vi "PH_OceanOpticsSpectrometer.ProcCases.vi"(0 "i ref in":refnum<vi>, 1 "selector":string, 2 "Data":T1, 3 "call cluster":T2={"Object"="", "Selector"="", "CallType"=enum."synchronous", "Async Object"="", "Async Selector"="", "Data Descriptor"="", "Data"=[], "Error #"=0, "Expire"=0}, 5 "error in (no error)":errorcluster) -> (14 "i ref out":refnum<vi>, 17 "answer cluster":T2={"Object"="", "Selector"="", "CallType"=enum."synchronous", "Async Object"="", "Async Selector"="", "Data Descriptor"="", "Data"=[], "Error #"=0, "Expire"=0}, 19 "error out":errorcluster)   [LabVIEW 2014, in "PH_OceanOpticsSpectrometer.lvlib"]
doc: "This method is called by a process from within the default case in the event loop. The methods of a class that are linked to events will be called from THIS method. Add your code here."
uses:
  PH_OceanOpticsSpectrometer.lvlib
  CS_Core/CSSystem/CoreDefs/CoreDefs.call_type.ctl
  CS_Core/BaseProcess/BaseProcess.descriptor string definition.ctl
  CS_Core/CSSystem/CoreDefs/CoreDefs.rawDataType.ctl
  CS_Core/CSSystem/CoreLib/CoreLib.byte array 2 short.vi
  CS_Core/CSSystem/CoreLib/CoreLib.string 2 byte array.vi
  CS_Core/CSSystem/CoreLib/CoreLib.byte array 2 double.vi
  CS_Core/BaseProcess/BaseProcess.lvlib
  CS_Core/CSSystem/CoreLib/CoreLib.lvlib
  CS_Core/CSSystem/CSSystemLib/CSSystemLib.lvlib
  CS_Core/CAEObj/CAEObj.lvlib
  PH_Basics/PH_PSDBWriter/PH_PSDBWriter.lvlib
  PH_Basics/PH_Common/PH_Common.lvlib
  PH_Basics/PH_StatusHandler/PH_StatusHandler.lvlib
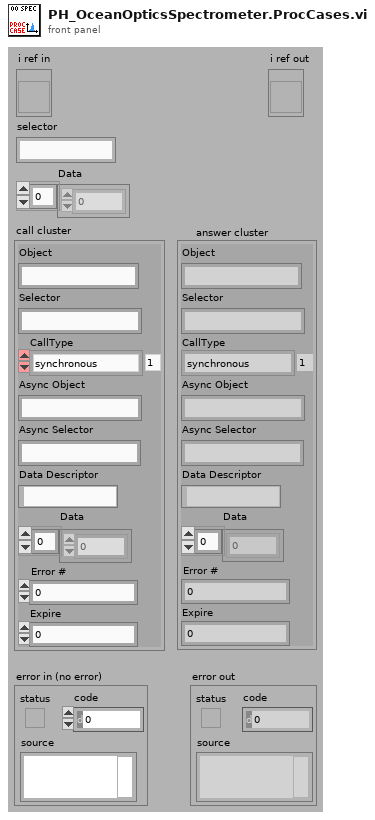
[diagram p1: front panel]
types:
  T1 = typedef "CoreDefs.rawDataType.ctl" = i8[]
  T2 = typedef "CoreDefs.call_type.ctl" = cluster{"Object":string, "Selector":string, "CallType":enum16{"simple", "synchronous", "asynchronous"}, "Async Object":string, "Async Selector":string, "Data Descriptor":T3, "Data":T1, "Error #":i32, "Expire":u32}
  T3 = typedef "BaseProcess.lvlib/BaseProcess.descriptor string definition.ctl" = string
  T4 = typedef "PH_OceanOpticsSpectrometer.lvlib/PH_OceanOpticsSpectrometer.i attribute.ctl" = cluster{"GUI Refs":cluster{"Delete":refnum<vi>, "Spectrum":refnum<vi>, "Display Width":refnum<vi>, "Display Center":refnum<vi>, "Save":refnum<vi>, "Integration time":refnum<vi>, "center wavelength":refnum<vi>, "width":refnum<vi>, "Wanted Trigger Mode":refnum<vi>, "Current Trigger Mode":refnum<vi>, "Trigger Info":refnum<vi>, "Model":refnum<vi>, "Driver":refnum<vi>, "Firmware":refnum<vi>}, "Display":cluster{"Width":dbl, "Center":dbl}, "VISA resource name":refnum<visa-resource-name>, "Integration time [ms]":cluster{"Current Value":u16, "Wanted Value":u16}, "Trigger":cluster{"Current value":T5, "Wanted value":T5}, "Default VISA Timeout":u32, "Last Data":cluster{"Wavelength Bins":dbl[], "Spectrum by Pixels":dbl[]}}
  T5 = typedef "PH_OceanOpticsSpectrometer.lvlib/PH_OceanOpticsSpectrometer.Trigger.ctl" = enum32{"External", "Normal"}
  T6 = typedef "PH_PSDBWriter.lvlib/PH_PSDBWriter.PHELIX-Subsystems.ctl" = i32
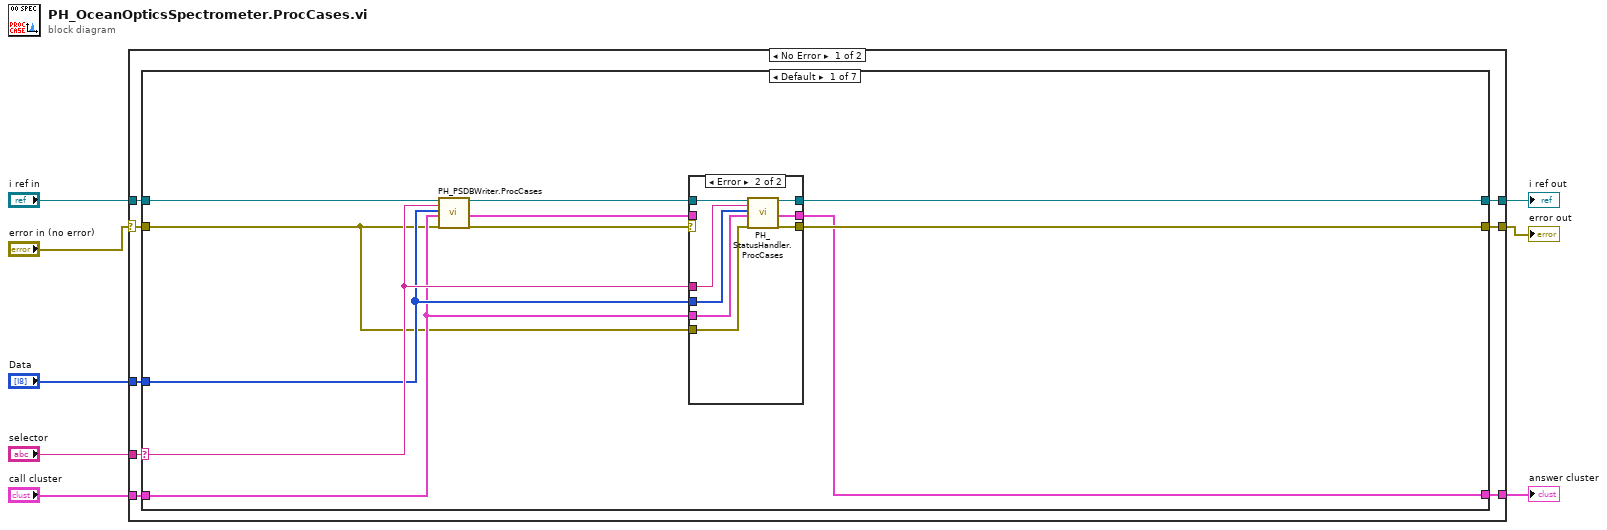
[diagram p0: block diagram]
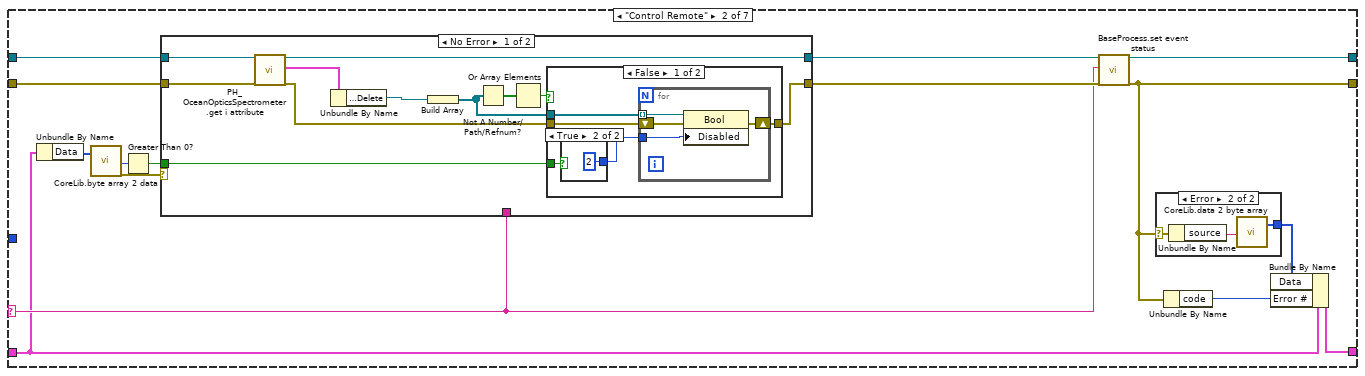
[diagram p3: hidden frame]
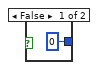
[diagram p5: hidden frame]
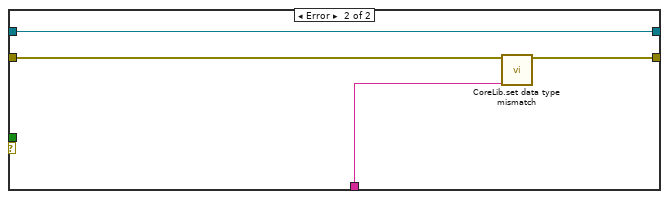
[diagram p7: hidden frame]
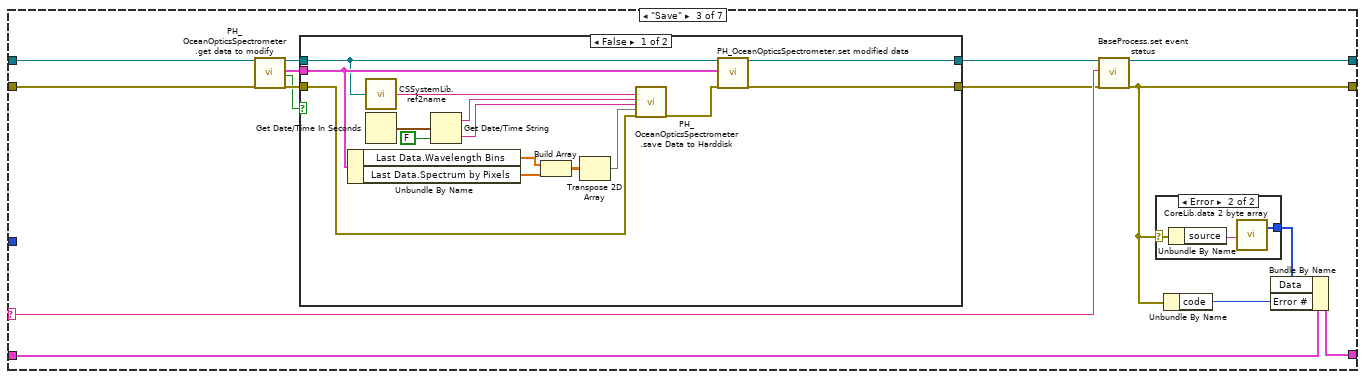
[diagram p8: hidden frame]
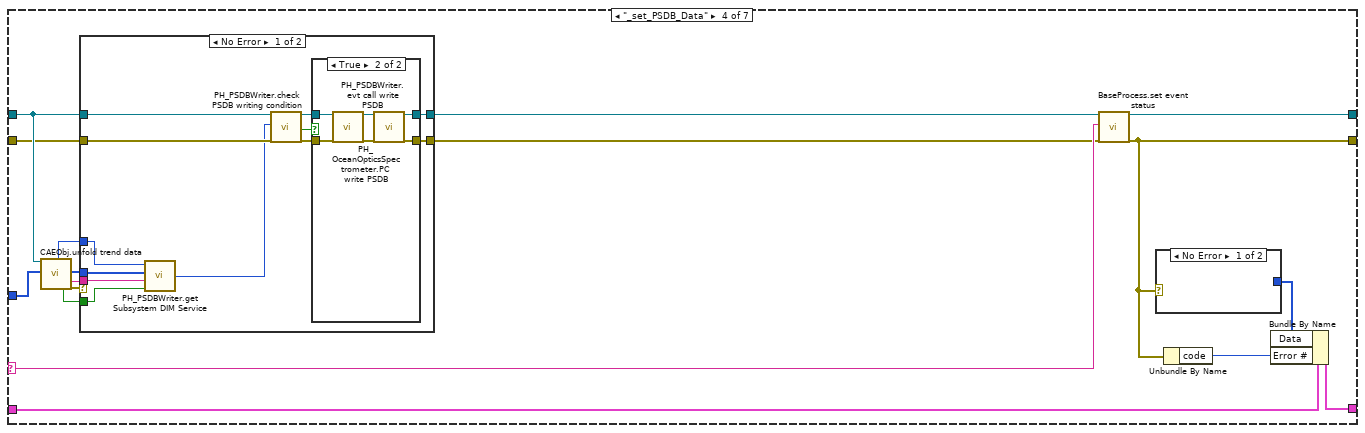
[diagram p11: hidden frame]
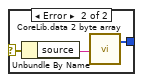
[diagram p14: hidden frame]
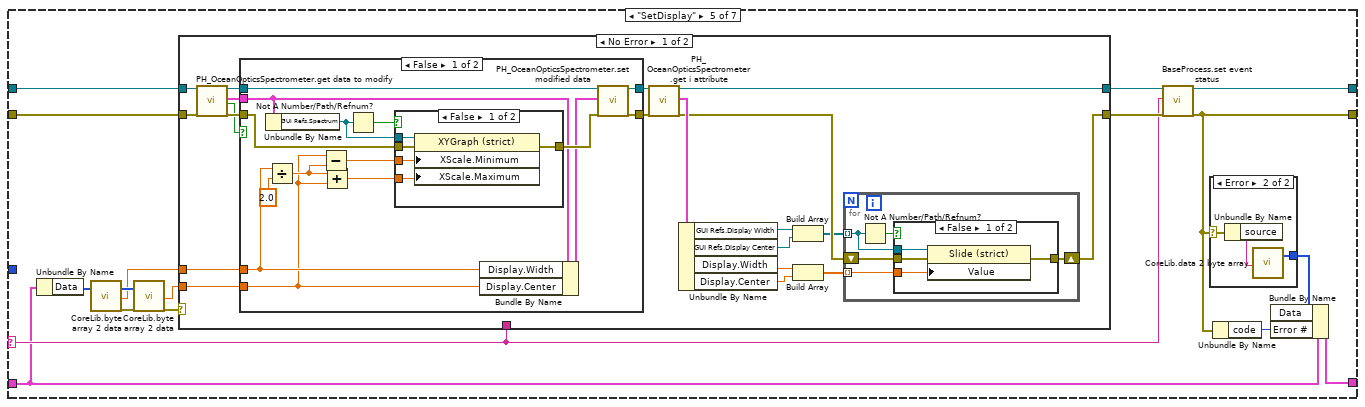
[diagram p15: hidden frame]
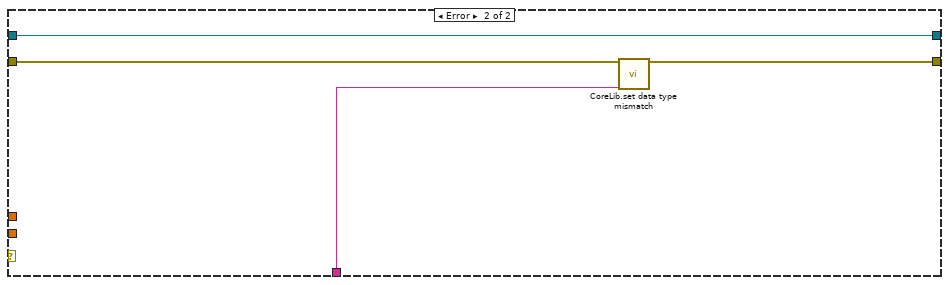
[diagram p20: hidden frame]
diagram:
  n1 = case shown="No Error" "error in (no error)" {
    selector: "error in (no error)" -> [w9 w333]
    tunnel: "selector" -> [w16 _]
    tunnel: [w15 w334] -> w7
    tunnel: "call cluster" -> [w14 w334]
    tunnel: "i ref in" -> [w13 w332]
    tunnel: [w12 w332] -> w4
    tunnel: [w11 w333] -> w3
    tunnel: "Data" -> [w10 _]
    frame No Error {
      n2 = case shown="Default" w16 {
        selector: w16 -> [w20 w50 w97 w135 w174 w248 w294]
        tunnel: w13 -> [w27 w48 w95 w127 w172 w246 w292]
        tunnel: [w24 w49 w96 w134 w173 w247 w293] -> w12
        tunnel: w14 -> [w18 w40 w91 w130 w167 w241 w287]
        tunnel: [w21 w39 w90 w129 w166 w240 w286] -> w15
        tunnel: w9 -> [w17 w53 w98 w126 w177 w251 w297]
        tunnel: [w23 w41 w92 w131 w168 w242 w288] -> w11
        tunnel: w10 -> [w19 _ _ w128 _ _ _]
        frame Default {
          n3 = call "PH_PSDBWriter.ProcCases.vi"("i ref in"=w27, "selector"=w20, "Data"=w19, "call cluster"=w18, "error in"=w17) -> ("i ref out"=w26:refnum<vi>, "answer cluster"=w22:T2, "error out"=w25:errorcluster)  [unwired: 12 in]
          n4 = case shown="Error" w25 {
            selector: w25 -> [w29 _]
            tunnel: [w29 w38] -> w23
            tunnel: w26 -> [w30 w37]
            tunnel: [w30 w36] -> w24
            tunnel: [w28 w35] -> w21
            tunnel: w17 -> [_ w34]
            tunnel: w18 -> [_ w33]
            tunnel: w19 -> [_ w32]
            tunnel: w20 -> [_ w31]
            tunnel: w22 -> [w28 _]
            frame No Error {
            }
            frame Error {
              n5 = call "PH_StatusHandler.ProcCases.vi"("i ref in"=w37, "selector"=w31, "Data"=w32, "call cluster"=w33, "error in (no error)"=w34) -> ("i ref out"=w36:refnum<vi>, "answer cluster"=w35:T2, "error out"=w38:errorcluster)  [unwired: 12 in]
            }
          }
        }
        frame "Control Remote" {
          n6 = Unbundle By Name(w40) -> ("Data"=w47:T1)
          n7 = call-poly "CoreLib.byte array 2 data.vi"("byteArray"=w47) -> ("i16"=w46:i16, "error out"=w44:errorcluster)  [unwired: 16 in, 1 out]
          n8 = Greater Than 0?(x=w46) -> (x > 0?=w45:bool)
          n9 = case shown="No Error" w44 {
            tunnel: [w63 w83] -> w52
            tunnel: w48 -> [w67 w83]
            tunnel: w53 -> [w66 w82]
            tunnel: [w62 w81] -> w51
            tunnel: w50 -> [_ w80]
            tunnel: w45 -> [w61 _]
            frame No Error {
              n10 = call "PH_OceanOpticsSpectrometer.get i attribute.vi"("i ref in"=w67, "error in (no error)"=w66) -> ("i ref out"=w63:refnum<vi>, "i attribute"=w65:T4, "error out"=w64:errorcluster)  [unwired: 15 in]
              n11 = Unbundle By Name(w65) -> ("GUI Refs.Delete"=w60:refnum<vi>)
              n12 = Build Array(w60) -> (w59:refnum<vi>[])
              n13 = Not A Number/Path/Refnum?(number/path/refnum=w59) -> (NaN/Path/Refnum?=w58:bool[])
              n14 = Or Array Elements(Boolean array=w58) -> (logical OR=w57:bool)
              n15 = case shown="False" w57 {
                tunnel: w59 -> [w72 _]
                tunnel: w64 -> [w71 w79]
                tunnel: [w70 w79] -> w62
                tunnel: w61 -> [w69 _]
                frame False {
                  n16 = case shown="True" w69 {
                    tunnel: [0 2] -> w68
                    frame False {
                    }
                    frame True {
                    }
                  }
                  n17 = for {
                    tunnel: w72 -> [w76] mode=indexing
                    tunnel: w68 -> [w73]
                    shift-right: [w74] -> w70
                    shift-left: w71 -> [w75]
                    n18 = property class="Bool"(reference=w76, error in=w75, "Disabled"=w73) -> (error out=w74:errorcluster)  [unwired: 1 out]
                  }
                }
                frame True {
                }
              }
            }
            frame Error {
              n19 = call "CoreLib.set data type mismatch.vi"("error in (no error)"=w82, "error source"=w80) -> ("error out"=w81:errorcluster)  [unwired: 17 in]
            }
          }
          n20 = call "BaseProcess.set event status.vi"("i ref in"=w52, "EventStatus"=w50, "error in (no error)"=w51) -> ("i ref out"=w49:refnum<vi>, "error out"=w41:errorcluster)  [unwired: 14 in, 1 out]
          n21 = case shown="Error" w41 {
            selector: w41 -> [_ w56]
            tunnel: [_ w54] -> w42
            frame No Error {
            }
            frame Error {
              n22 = Unbundle By Name(w56) -> ("source"=w55:string)
              n23 = call-poly "CoreLib.data 2 byte array.vi"("string"=w55) -> ("byteArray out"=w54:T1)  [unwired: 18 in]
            }
          }
          n24 = Unbundle By Name(w41) -> ("code"=w43:i32)
          n25 = Bundle By Name(cluster=w40, "Data"=w42, "Error #"=w43) -> (w39:T2)
        }
        frame "Save" {
          n26 = call "PH_OceanOpticsSpectrometer.get data to modify.vi"("i ref in"=w95, "error in (no error)"=w98) -> ("i ref out"=w89:refnum<vi>, "i attribute"=w84:T4, "timed out"=w85:bool, "error out"=w87:errorcluster)  [unwired: 14 in]
          n27 = case shown="False" w85 {
            tunnel: w89 -> [w111 w115]
            tunnel: [w113 w115] -> w88
            tunnel: w87 -> [w103 w114]
            tunnel: [w105 w114] -> w86
            tunnel: w84 -> [w112 _]
            frame False {
              n28 = Unbundle By Name(w112) -> ("Last Data.Wavelength Bins"=w100:dbl[], "Last Data.Spectrum by Pixels"=w101:dbl[])
              n29 = call "CSSystemLib.ref2name.vi"("obj refnum"=w111) -> ("name"=w110:string)
              n30 = Get Date/Time In Seconds() -> (seconds since 1Jan1904=w108:timestamp)
              n31 = Get Date/Time String(seconds (now)=w108, want seconds? (F)=FALSE) -> (date string=w107:string, time string=w106:string)  [unwired: 1 in]
              n32 = Build Array(w100, w101) -> (w102:dbl[][])
              n33 = Transpose 2D Array(2D array=w102) -> (transposed array=w99:dbl[][])
              n34 = call "PH_OceanOpticsSpectrometer.save Data to Harddisk.vi"("Instance name"=w110, "Recording Date"=w107, "Recording Time"=w106, "Data"=w99, "error in"=w103) -> ("error out"=w104:errorcluster)  [unwired: 14 in]
              n35 = call "PH_OceanOpticsSpectrometer.set modified data.vi"("i ref in"=w111, "i attribute"=w112, "error in (no error)"=w104) -> ("i ref out"=w113:refnum<vi>, "error out"=w105:errorcluster)  [unwired: 15 in]
            }
            frame True {
            }
          }
          n36 = call "BaseProcess.set event status.vi"("i ref in"=w88, "EventStatus"=w97, "error in (no error)"=w86) -> ("i ref out"=w96:refnum<vi>, "error out"=w92:errorcluster)  [unwired: 14 in, 1 out]
          n37 = case shown="Error" w92 {
            selector: w92 -> [_ w118]
            tunnel: [_ w116] -> w93
            frame No Error {
            }
            frame Error {
              n38 = Unbundle By Name(w118) -> ("source"=w117:string)
              n39 = call-poly "CoreLib.data 2 byte array.vi"("string"=w117) -> ("byteArray out"=w116:T1)  [unwired: 18 in]
            }
          }
          n40 = Unbundle By Name(w92) -> ("code"=w94:i32)
          n41 = Bundle By Name(cluster=w91, "Data"=w93, "Error #"=w94) -> (w90:T2)
        }
        frame "_set_PSDB_Data" {
          n42 = call "CAEObj.unfold trend data.vi"("i ref in"=w127, "raw trend data"=w128) -> ("quality"=w121:i32, "no link"=w122:bool, "data"=w120:i8[], "typeDescriptor"=w119:string, "error out"=w123:errorcluster)  [unwired: 9 in, 4 out]
          n43 = case shown="No Error" w123 {
            tunnel: w126 -> [w147 w157]
            tunnel: [w146 w156] -> w125
            tunnel: [w145 w157] -> w124
            tunnel: w127 -> [w143 w156]
            tunnel: w122 -> [w138 _]
            tunnel: w119 -> [w139 _]
            tunnel: w120 -> [w140 _]
            tunnel: w121 -> [w137 _]
            frame No Error {
              n44 = call "PH_PSDBWriter.get Subsystem DIM Service.vi"("no link"=w138, "typeDescriptor"=w139, "data"=w140, "quality"=w137) -> ("PHELIX Subsystems"=w136:T6)
              n45 = call "PH_PSDBWriter.check PSDB writing condition.vi"("i ref in"=w143, "wanted Subsystem"=w136, "error IO"=w147) -> ("i ref out"=w142:refnum<vi>, "write PSDB?"=w141:bool, "error out"=w144:errorcluster)  [unwired: 14 in]
              n46 = case shown="True" w141 {
                tunnel: w144 -> [w148 w155]
                tunnel: [w149 w152] -> w146
                tunnel: [w148 w150] -> w145
                tunnel: w142 -> [w149 w154]
                frame False {
                }
                frame True {
                  n47 = call "PH_OceanOpticsSpectrometer.PC write PSDB.vi"("i ref in"=w154, "error IO"=w155) -> ("i ref out"=w153:refnum<vi>, "error out"=w151:errorcluster)  [unwired: 16 in]
                  n48 = call "PH_PSDBWriter.evt call write PSDB.vi"("i ref in"=w153, "error in (no error)"=w151) -> ("i ref out"=w152:refnum<vi>, "error out"=w150:errorcluster)  [unwired: 16 in]
                }
              }
            }
            frame Error {
            }
          }
          n49 = call "BaseProcess.set event status.vi"("i ref in"=w125, "EventStatus"=w135, "error in (no error)"=w124) -> ("i ref out"=w134:refnum<vi>, "error out"=w131:errorcluster)  [unwired: 14 in, 1 out]
          n50 = case shown="No Error" w131 {
            selector: w131 -> [_ w160]
            tunnel: [_ w158] -> w132
            frame No Error {
            }
            frame Error {
              n51 = Unbundle By Name(w160) -> ("source"=w159:string)
              n52 = call-poly "CoreLib.data 2 byte array.vi"("string"=w159) -> ("byteArray out"=w158:T1)  [unwired: 18 in]
            }
          }
          n53 = Unbundle By Name(w131) -> ("code"=w133:i32)
          n54 = Bundle By Name(cluster=w130, "Data"=w132, "Error #"=w133) -> (w129:T2)
        }
        frame "SetDisplay" {
          n55 = Unbundle By Name(w167) -> ("Data"=w171:T1)
          n56 = call-poly "CoreLib.byte array 2 data.vi"("byteArray"=w171) -> ("byteArray out"=w163:T1, "d64"=w162:dbl, "error out"=w165:errorcluster)  [unwired: 16 in]
          n57 = call-poly "CoreLib.byte array 2 data.vi"("byteArray"=w163, "error in (no error)"=w165) -> ("d64"=w161:dbl, "error out"=w164:errorcluster)  [unwired: 15 in, 1 out]
          n58 = case shown="No Error" w164 {
            tunnel: [w191 w237] -> w176
            tunnel: w172 -> [w200 w237]
            tunnel: w177 -> [w199 w236]
            tunnel: [w183 w235] -> w175
            tunnel: w174 -> [_ w234]
            tunnel: w162 -> [w194 _]
            tunnel: w161 -> [w193 _]
            frame No Error {
              n59 = call "PH_OceanOpticsSpectrometer.get data to modify.vi"("i ref in"=w200, "error in (no error)"=w199) -> ("i ref out"=w197:refnum<vi>, "i attribute"=w198:T4, "timed out"=w195:bool, "error out"=w196:errorcluster)  [unwired: 14 in]
              n60 = case shown="False" w195 {
                tunnel: w198 -> [w214 _]
                tunnel: w197 -> [w225 w233]
                tunnel: [w224 w233] -> w190
                tunnel: w196 -> [w218 w232]
                tunnel: [w223 w232] -> w192
                tunnel: w194 -> [w212 _]
                tunnel: w193 -> [w211 _]
                frame False {
                  n61 = Unbundle By Name(w214) -> ("GUI Refs.Spectrum"=w215:refnum<vi>)
                  n62 = Divide(x=w212, y=2.0) -> (x/y=w221:dbl)
                  n63 = Subtract(x=w211, y=w221) -> (x-y=w220:dbl)
                  n64 = Add(x=w221, y=w211) -> (x+y=w219:dbl)
                  n65 = Not A Number/Path/Refnum?(number/path/refnum=w215) -> (NaN/Path/Refnum?=w216:bool)
                  n66 = case shown="False" w216 {
                    tunnel: w215 -> [w230 _]
                    tunnel: w220 -> [w229 _]
                    tunnel: w219 -> [w228 _]
                    tunnel: w218 -> [w227 w231]
                    tunnel: [w226 w231] -> w217
                    frame False {
                      n67 = property on="Property Node" class="XYGraph (strict)"(reference=w230, error in=w227, "XScale.Minimum"=w229, "XScale.Maximum"=w228) -> (error out=w226:errorcluster)  [unwired: 1 out]
                    }
                    frame True {
                    }
                  }
                  n68 = Bundle By Name(cluster=w214, "Display.Width"=w212, "Display.Center"=w211) -> (w213:T4)
                  n69 = call "PH_OceanOpticsSpectrometer.set modified data.vi"("i ref in"=w225, "i attribute"=w213, "error in (no error)"=w217) -> ("i ref out"=w224:refnum<vi>, "error out"=w223:errorcluster)  [unwired: 15 in]
                }
                frame True {
                }
              }
              n70 = call "PH_OceanOpticsSpectrometer.get i attribute.vi"("i ref in"=w190, "error in (no error)"=w192) -> ("i ref out"=w191:refnum<vi>, "i attribute"=w189:T4, "error out"=w184:errorcluster)  [unwired: 15 in]
              n71 = Unbundle By Name(w189) -> ("GUI Refs.Display Width"=w186:refnum<vi>, "GUI Refs.Display Center"=w185:refnum<vi>, "Display.Width"=w188:dbl, "Display.Center"=w187:dbl)
              n72 = Build Array(w186, w185) -> (w182:refnum<vi>[])
              n73 = Build Array(w188, w187) -> (w181:dbl[])
              n74 = for {
                shift-right: [w203] -> w183
                shift-left: w184 -> [w204]
                tunnel: w182 -> [w202] mode=indexing
                tunnel: w181 -> [w201] mode=indexing
                n75 = Not A Number/Path/Refnum?(number/path/refnum=w202) -> (NaN/Path/Refnum?=w205:bool)
                n76 = case shown="False" w205 {
                  tunnel: w202 -> [w208 _]
                  tunnel: w204 -> [w209 w210]
                  tunnel: [w207 w210] -> w203
                  tunnel: w201 -> [w206 _]
                  frame False {
                    n77 = property class="Slide (strict)"(reference=w208, error in=w209, "Value"=w206) -> (error out=w207:errorcluster)  [unwired: 1 out]
                  }
                  frame True {
                  }
                }
              }
            }
            frame Error {
              n78 = call "CoreLib.set data type mismatch.vi"("error in (no error)"=w236, "error source"=w234) -> ("error out"=w235:errorcluster)  [unwired: 17 in]
            }
          }
          n79 = call "BaseProcess.set event status.vi"("i ref in"=w176, "EventStatus"=w174, "error in (no error)"=w175) -> ("i ref out"=w173:refnum<vi>, "error out"=w168:errorcluster)  [unwired: 14 in, 1 out]
          n80 = case shown="Error" w168 {
            selector: w168 -> [_ w180]
            tunnel: [_ w178] -> w169
            frame No Error {
            }
            frame Error {
              n81 = Unbundle By Name(w180) -> ("source"=w179:string)
              n82 = call-poly "CoreLib.data 2 byte array.vi"("string"=w179) -> ("byteArray out"=w178:T1)  [unwired: 18 in]
            }
          }
          n83 = Unbundle By Name(w168) -> ("code"=w170:i32)
          n84 = Bundle By Name(cluster=w167, "Data"=w169, "Error #"=w170) -> (w166:T2)
        }
        frame "SetIntegrationTime" {
          n85 = Unbundle By Name(w241) -> ("Data"=w245:T1)
          n86 = call-poly "CoreLib.byte array 2 data.vi"("byteArray"=w245) -> ("i16"=w239:i16, "error out"=w238:errorcluster)  [unwired: 16 in, 1 out]
          n87 = case shown="No Error" w238 {
            tunnel: [w256 w283] -> w250
            tunnel: w246 -> [w263 w283]
            tunnel: w251 -> [w262 w282]
            tunnel: [w255 w281] -> w249
            tunnel: w248 -> [_ w280]
            tunnel: w239 -> [w257 _]
            frame No Error {
              n88 = call "PH_OceanOpticsSpectrometer.get data to modify.vi"("i ref in"=w263, "error in (no error)"=w262) -> ("i ref out"=w260:refnum<vi>, "i attribute"=w261:T4, "timed out"=w258:bool, "error out"=w259:errorcluster)  [unwired: 14 in]
              n89 = case shown="False" w258 {
                tunnel: w261 -> [w276 _]
                tunnel: w260 -> [w277 w279]
                tunnel: [w272 w279] -> w256
                tunnel: w259 -> [w265 w278]
                tunnel: [w273 w278] -> w255
                tunnel: w257 -> [w274 _]
                frame False {
                  n90 = To Unsigned Word Integer(number=w274) -> (unsigned 16bit integer=w271:u16)
                  n91 = Unbundle By Name(w276) -> ("GUI Refs.Integration time"=w267:refnum<vi>, "Integration time [ms].Current Value"=w266:u16)
                  n92 = In Range and Coerce(upper limit=u16 500, x=w271, lower limit=u16 1) -> (coerced(x)=w270:u16)  [unwired: 1 out]
                  n93 = Bundle By Name(cluster=w276, "Integration time [ms].Wanted Value"=w270) -> (w275:T4)
                  n94 = call "PH_GUI.set U16 GUI object.vi"("U16 Ref"=w267, "Value"=w266, "error in (no error)"=w265) -> ("error out"=w264:errorcluster)  [unwired: 16 in]
                  n95 = call "PH_OceanOpticsSpectrometer.set modified data.vi"("i ref in"=w277, "i attribute"=w275, "error in (no error)"=w264) -> ("i ref out"=w272:refnum<vi>, "error out"=w273:errorcluster)  [unwired: 15 in]
                }
                frame True {
                }
              }
            }
            frame Error {
              n96 = call "CoreLib.set data type mismatch.vi"("error in (no error)"=w282, "error source"=w280) -> ("error out"=w281:errorcluster)  [unwired: 17 in]
            }
          }
          n97 = call "BaseProcess.set event status.vi"("i ref in"=w250, "EventStatus"=w248, "error in (no error)"=w249) -> ("i ref out"=w247:refnum<vi>, "error out"=w242:errorcluster)  [unwired: 14 in, 1 out]
          n98 = case shown="Error" w242 {
            selector: w242 -> [_ w254]
            tunnel: [_ w252] -> w243
            frame No Error {
            }
            frame Error {
              n99 = Unbundle By Name(w254) -> ("source"=w253:string)
              n100 = call-poly "CoreLib.data 2 byte array.vi"("string"=w253) -> ("byteArray out"=w252:T1)  [unwired: 18 in]
            }
          }
          n101 = Unbundle By Name(w242) -> ("code"=w244:i32)
          n102 = Bundle By Name(cluster=w241, "Data"=w243, "Error #"=w244) -> (w240:T2)
        }
        frame "SetTriggerMode" {
          n103 = Unbundle By Name(w287) -> ("Data"=w291:T1)
          n104 = call-poly "CoreLib.byte array 2 data.vi"("byteArray"=w291) -> ("i16"=w285:i16, "error out"=w284:errorcluster)  [unwired: 16 in, 1 out]
          n105 = case shown="No Error" w284 {
            tunnel: [w302 w331] -> w296
            tunnel: w292 -> [w309 w331]
            tunnel: w297 -> [w308 w330]
            tunnel: [w301 w329] -> w295
            tunnel: w294 -> [_ w328]
            tunnel: w285 -> [w303 _]
            frame No Error {
              n106 = call "PH_OceanOpticsSpectrometer.get data to modify.vi"("i ref in"=w309, "error in (no error)"=w308) -> ("i ref out"=w306:refnum<vi>, "i attribute"=w307:T4, "timed out"=w304:bool, "error out"=w305:errorcluster)  [unwired: 14 in]
              n107 = case shown="False" w304 {
                tunnel: w307 -> [w317 _]
                tunnel: w306 -> [w320 w327]
                tunnel: [w319 w327] -> w302
                tunnel: w305 -> [w313 w326]
                tunnel: [w318 w326] -> w301
                tunnel: w303 -> [w311 _]
                frame False {
                  n108 = Unbundle By Name(w317) -> ("GUI Refs.Wanted Trigger Mode"=w314:refnum<vi>)
                  n109 = To Unsigned Long Integer(number=w311) -> (unsigned 32bit integer=w310:u32)
                  n110 = Not A Number/Path/Refnum?(number/path/refnum=w314) -> (NaN/Path/Refnum?=w315:bool)
                  n111 = case shown="False" w315 {
                    tunnel: w314 -> [w324 _]
                    tunnel: w313 -> [w323 w325]
                    tunnel: [w322 w325] -> w312
                    tunnel: w310 -> [w321 _]
                    frame False {
                      n112 = property class="RadioBtnsControl (strict)"(reference=w324, error in=w323, "Value"=w321) -> (error out=w322:errorcluster)  [unwired: 1 out]
                    }
                    frame True {
                    }
                  }
                  n113 = Bundle By Name(cluster=w317, "Trigger.Wanted value"=w310) -> (w316:T4)
                  n114 = call "PH_OceanOpticsSpectrometer.set modified data.vi"("i ref in"=w320, "i attribute"=w316, "error in (no error)"=w312) -> ("i ref out"=w319:refnum<vi>, "error out"=w318:errorcluster)  [unwired: 15 in]
                }
                frame True {
                }
              }
            }
            frame Error {
              n115 = call "CoreLib.set data type mismatch.vi"("error in (no error)"=w330, "error source"=w328) -> ("error out"=w329:errorcluster)  [unwired: 17 in]
            }
          }
          n116 = call "BaseProcess.set event status.vi"("i ref in"=w296, "EventStatus"=w294, "error in (no error)"=w295) -> ("i ref out"=w293:refnum<vi>, "error out"=w288:errorcluster)  [unwired: 14 in, 1 out]
          n117 = case shown="Error" w288 {
            selector: w288 -> [_ w300]
            tunnel: [_ w298] -> w289
            frame No Error {
            }
            frame Error {
              n118 = Unbundle By Name(w300) -> ("source"=w299:string)
              n119 = call-poly "CoreLib.data 2 byte array.vi"("string"=w299) -> ("byteArray out"=w298:T1)  [unwired: 18 in]
            }
          }
          n120 = Unbundle By Name(w288) -> ("code"=w290:i32)
          n121 = Bundle By Name(cluster=w287, "Data"=w289, "Error #"=w290) -> (w286:T2)
        }
      }
    }
    frame Error {
    }
  }
  "answer cluster" <- w7
  "i ref out" <- w4
  "error out" <- w3
